vi "Write Introspection Output.vi"(8 "error in (no error)":errorcluster, 10 "Introspection":T1, 11 "ONNX Class in":refnum<class "ONNX Class.lvclass">) -> (0 "error out":errorcluster, 3 "ONNX Class out":refnum<class "ONNX Class.lvclass">)   [LabVIEW 2017, in "ONNX Class Library.lvlib" / "ONNX Class.lvclass"]
uses:
  ONNX Class.lvclass
  ONNX Class.lvclass/ONNX Class.ctl
  TypeDef/IO.ctl
  ONNX Class Library.lvlib
  TypeDef/Introspection.ctl
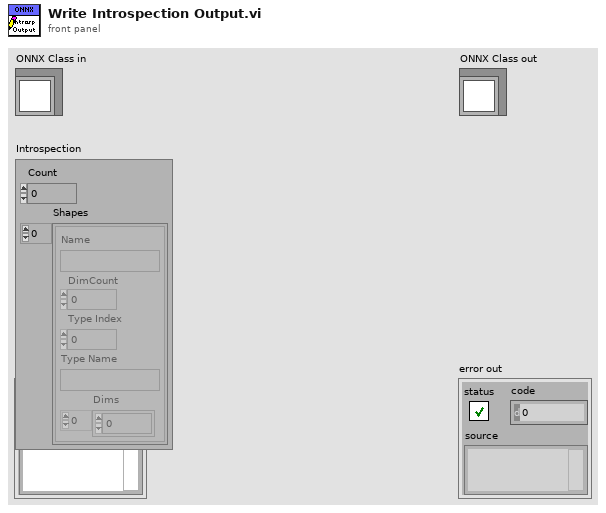
[diagram p1: front panel]
types:
  T1 = typedef "ONNX Class Library.lvlib/Introspection.ctl" = cluster{"Count":i32, "Shapes":T2[]}
  T2 = typedef "ONNX Class Library.lvlib/IO.ctl" = cluster{"Name":string, "DimCount":i32, "Type Index":i32, "Type Name":string, "Dims":i64[]}
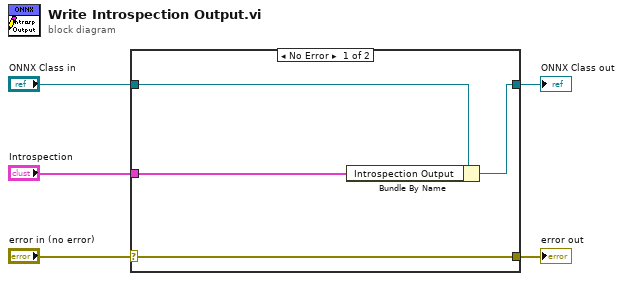
[diagram p0: block diagram]
diagram:
  n1 = case shown="No Error" "error in (no error)" {
    selector: "error in (no error)" -> [w9 w10]
    tunnel: [w9 w10] -> w4
    tunnel: [w7 w11] -> w2
    tunnel: "ONNX Class in" -> [w8 w11]
    tunnel: "Introspection" -> [w6 _]
    frame No Error {
      n2 = Bundle By Name(cluster=w8, "Introspection Output"=w6) -> (w7:refnum<class "ONNX Class.lvclass">)
    }
    frame Error {
    }
  }
  "error out" <- w4
  "ONNX Class out" <- w2
